vi "osa_get measurement command string.vi"(2 "precision (Hz)":dbl, 3 "HS frequency (Hz)":dbl, 4 "OS frequency (Hz)":dbl) -> (0 "status string":string, 1 "command string":string)   [LabVIEW 2021]
panel:
  # "OSA subVI: convert OS/HS frequency settings to serial command and status string"
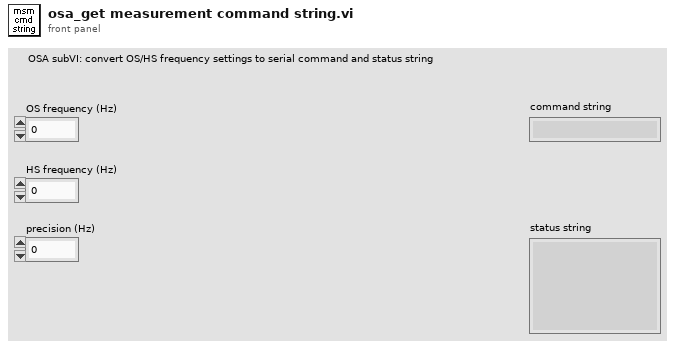
[diagram p1: front panel]
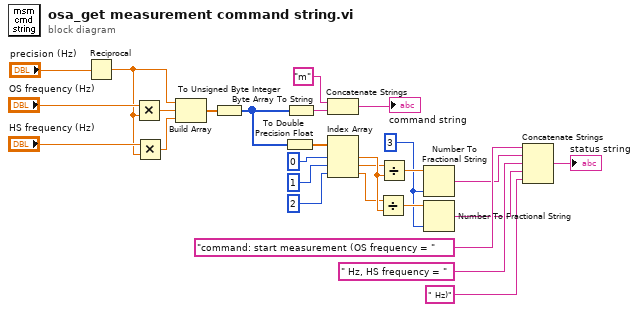
[diagram p0: block diagram]
diagram:
  w1 = i16 3
  n1 = Reciprocal(x="precision (Hz)") -> (1/x=w5:dbl)
  n2 = Multiply(x="OS frequency (Hz)", y=w5) -> (x*y=w27:dbl)
  n3 = Multiply(x="HS frequency (Hz)", y=w5) -> (x*y=w26:dbl)
  n4 = Build Array(w5, w27, w26) -> (w25:dbl[])
  n5 = To Unsigned Byte Integer(number=w25) -> (unsigned 8bit integer=w18:u8[])
  n6 = To Double Precision Float(number=w18) -> (double precision float=w17:dbl[])
  n7 = Byte Array To String(unsigned byte array=w18) -> (string=w24:string)
  n8 = Concatenate Strings("m", w24) -> (→"command string":string)
  n9 = Index Array(array=w17, index #1=0, index #2=1, index #3=2) -> (element #1=w4:dbl, element #2=w3:dbl, element #3=w2:dbl)
  n10 = Divide(x=w2, y=w4) -> (x/y=w12:dbl)
  n11 = Divide(x=w3, y=w4) -> (x/y=w13:dbl)
  n12 = Number To Fractional String(number=w13, precision (6)=w1) -> (F-format string=w10:string)  [unwired: 2 in]
  n13 = Number To Fractional String(number=w12, precision (6)=w1) -> (F-format string=w8:string)  [unwired: 2 in]
  n14 = Concatenate Strings("command: start measurement (OS frequency = ", w10, " Hz, HS frequency = ", w8, " Hz)") -> (→"status string":string)
